vi "cube vision timed.vi"() -> ()   [LabVIEW 2017]
uses:
  <vilib>/vision/NI_Vision_Development_Module.lvlib
panel:
  out "trim image":u32=1
  out "fps":dbl=40.0
  out "total time":u32=25
  out "to 3D array":u32=6
  out "calc angle":u32
  out "threshhold":u32
  out "isolate green":u32=18
  out "to RGB array":u32=1
  out "angle":dbl=-14.305551846621954
  out "Color":T1(plugin-control)
  out "Binary Image":T1(plugin-control)
  in  "Sat Range":cluster{u8, u8}(slide)={255, 160} scale=0.0..255.0
  in  "Hue Range":cluster{u8, u8}(slide)={87, 19} scale=0.0..255.0
  in  "File Path":path=path "F:/power cube pics/5.bmp"
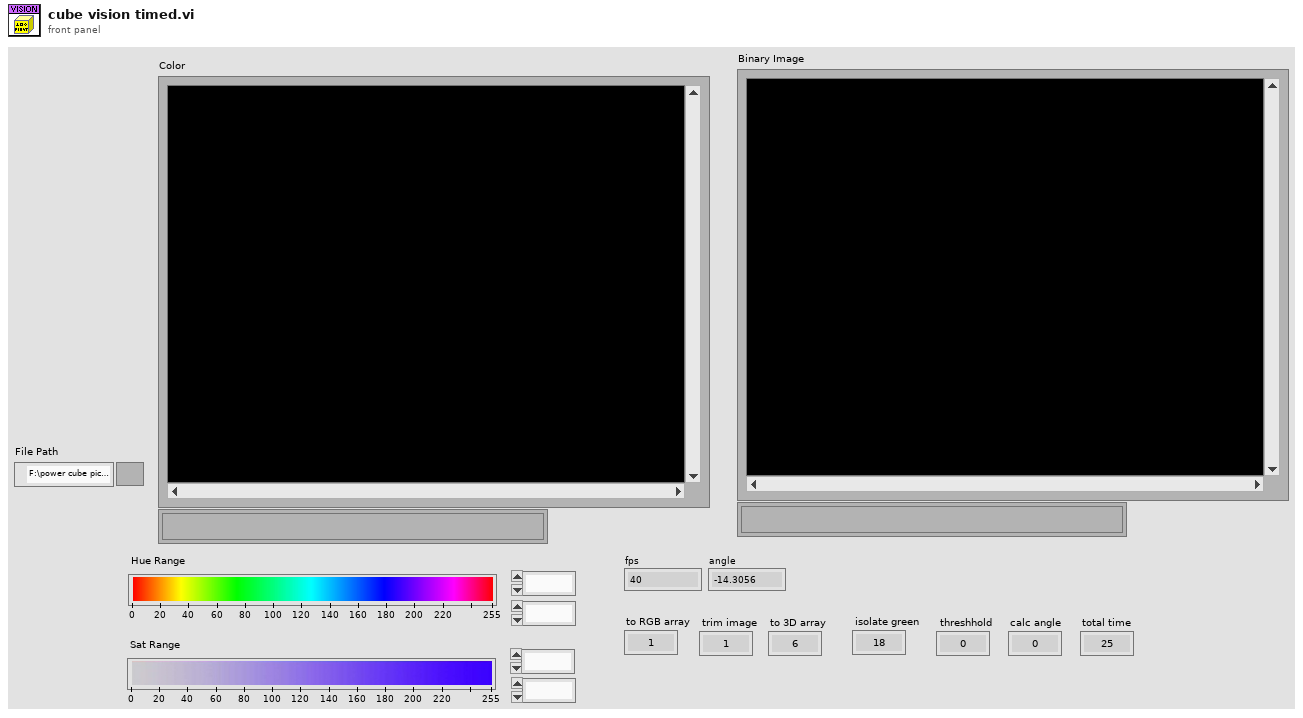
[diagram p1: front panel]
types:
  T1 = typedef "IMAQ Image.ctl" = refnum<image>
  T2 = typedef "Image Type" = u32
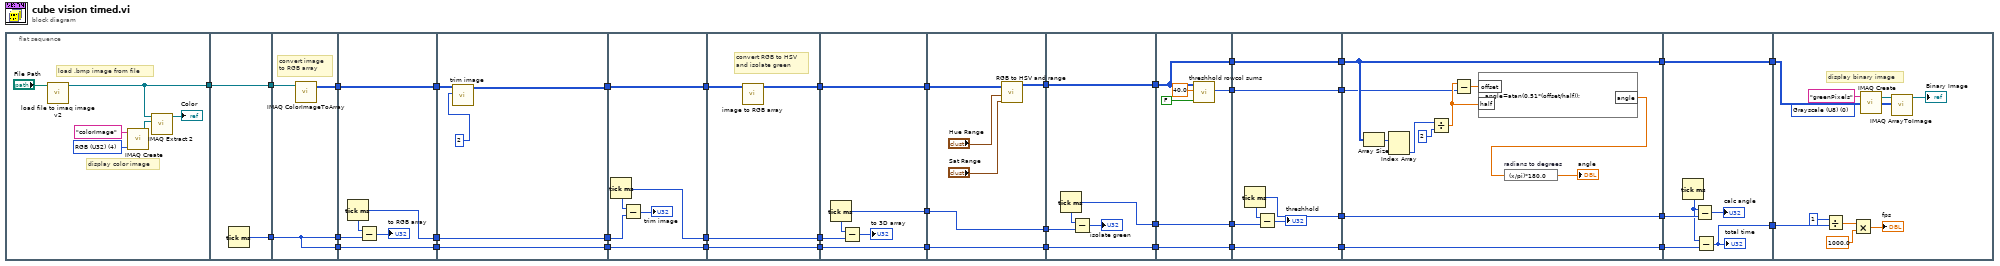
[diagram p0: block diagram]
diagram:
  n1 = flat-sequence {
    tunnel: [w42] -> w40
    tunnel: w40 -> [w48]
    tunnel: [w48] -> w39
    tunnel: [w47] -> w29
    tunnel: w39 -> [w51]
    tunnel: [w50] -> w38
    tunnel: [w49] -> w30
    tunnel: w29 -> [w49]
    tunnel: [w49] -> w18
    tunnel: w38 -> [w56]
    tunnel: [w56] -> w9
    tunnel: w30 -> [w55]
    tunnel: [w53] -> w8
    tunnel: w18 -> [w52]
    tunnel: [w52] -> w7
    tunnel: w9 -> [w59]
    tunnel: [w57] -> w6
    tunnel: w8 -> [w61]
    tunnel: [w61] -> w4
    tunnel: w7 -> [w60]
    tunnel: [w60] -> w2
    tunnel: w6 -> [w66]
    tunnel: [w66] -> w5
    tunnel: w4 -> [w63]
    tunnel: [w62] -> w3
    tunnel: w2 -> [w65]
    tunnel: [w65] -> w1
    tunnel: w5 -> [w70]
    tunnel: [w69] -> w22
    tunnel: w3 -> [w68]
    tunnel: [w68] -> w21
    tunnel: w1 -> [w67]
    tunnel: [w67] -> w17
    tunnel: [w75] -> w23
    tunnel: w22 -> [w75]
    tunnel: w21 -> [w73]
    tunnel: [w72] -> w19
    tunnel: w17 -> [w71]
    tunnel: [w71] -> w16
    tunnel: [w79] -> w24
    tunnel: w23 -> [w78]
    tunnel: [w77] -> w20
    tunnel: w19 -> [w77]
    tunnel: w16 -> [w76]
    tunnel: [w76] -> w15
    tunnel: w24 -> [w86]
    tunnel: [w86] -> w37
    tunnel: [w84] -> w27
    tunnel: w20 -> [w83]
    tunnel: w15 -> [w82]
    tunnel: [w82] -> w14
    tunnel: w37 -> [w92]
    tunnel: [w92] -> w36
    tunnel: [w89] -> w34
    tunnel: [w88] -> w28
    tunnel: w27 -> [w88]
    tunnel: w14 -> [w87]
    tunnel: [w87] -> w13
    tunnel: w36 -> [w98]
    tunnel: [w98] -> w35
    tunnel: w34 -> [w97]
    tunnel: [w97] -> w33
    tunnel: w28 -> [w95]
    tunnel: [w94] -> w26
    tunnel: w13 -> [w93]
    tunnel: [w93] -> w12
    tunnel: w35 -> [w109]
    tunnel: w33 -> [w104]
    tunnel: [w109] -> w32
    tunnel: w26 -> [w100]
    tunnel: [w100] -> w25
    tunnel: w12 -> [w99]
    tunnel: [w99] -> w11
    tunnel: w32 -> [w115]
    tunnel: [w115] -> w31
    tunnel: w25 -> [w113]
    tunnel: w11 -> [w111]
    tunnel: [w110] -> w10
    tunnel: w31 -> [w121]
    tunnel: w10 -> [w120]
    frame #0 {
      w44 = T2 4 items=["Grayscale (U8)", "Grayscale (I16)", "Grayscale (SGL)", "Complex (CSG)", "RGB (U32)", "HSL (U32)", "RGB (U64)", "Grayscale (U16)"] ("Image Type")
      # "display color image"
      # "load .bmp image from file"
      n2 = call "load file to imaq image v2.vi"("path to BMP file"="File Path") -> ("Image"=w42:T1)  [unwired: 9 in, 1 out]
      n3 = call "IMAQ Create"("Image Name"="colorImage", "Image Type"=w44) -> ("New Image"=w46:T1)  [unwired: 3 in, 1 out]
      n4 = call "IMAQ Extract 2"("Image Dst"=w46, "Image Src"=w42) -> ("Image Dst Out"=→"Color":T1)  [unwired: 8 in, 1 out]
    }
    frame #1 {
      n5 = Tick Count (ms)() -> (millisecond timer value=w47:u32)
    }
    frame #2 {
      # "convert image\nto RGB array"
      n6 = call "IMAQ ColorImageToArray"("Image"=w51) -> ("Image Pixels (U32)"=w50:u32[][])  [unwired: 3 in, 2 out]
    }
    frame #3 {
      n7 = Tick Count (ms)() -> (millisecond timer value=w53:u32)
      n8 = Subtract(x=w53, y=w55) -> (x-y=→"to RGB array":u32)
    }
    frame #4 {
      n9 = call "trim image.vi"("scale"=2, "Image Pixels (U32)"=w59) -> ("Trimmed Image Pixels (U32)"=w57:u32[][])  [unwired: 9 in]
    }
    frame #5 {
      n10 = Tick Count (ms)() -> (millisecond timer value=w62:u32)
      n11 = Subtract(x=w62, y=w63) -> (x-y=→"trim image":u32)
    }
    frame #6 {
      # "convert RGB to HSV\nand isolate green"
      n12 = call "image to RGB array.vi"("Image Pixels (U32)"=w70) -> ("Image Pixels (U8)"=w69:u8[][][])  [unwired: 10 in]
    }
    frame #7 {
      n13 = Tick Count (ms)() -> (millisecond timer value=w72:u32)
      n14 = Subtract(x=w72, y=w73) -> (x-y=→"to 3D array":u32)
    }
    frame #8 {
      n15 = call "RGB to HSV and range.vi"("Image Pixels (RGB)"=w78, "Hue Range"="Hue Range", "Sat Range"="Sat Range") -> ("Threshholded Pixels"=w79:u8[][])  [unwired: 7 in]
    }
    frame #9 {
      n16 = Tick Count (ms)() -> (millisecond timer value=w84:u32)
      n17 = Subtract(x=w84, y=w83) -> (x-y=→"isolate green":u32)
    }
    frame #10 {
      n18 = call "threshhold rowcol sums.vi"("Row(T)/Col(F)"=FALSE, "Threshold"=40.0, "Pixels"=w92) -> ("middle row/col"=w89:i32)  [unwired: 6 in, 2 out]
    }
    frame #11 {
      n19 = Tick Count (ms)() -> (millisecond timer value=w94:u32)
      n20 = Subtract(x=w94, y=w95) -> (x-y=→"threshhold":u32)
    }
    frame #12 {
      n21 = Array Size(array=w109) -> (size(s)=w105:i32[])
      n22 = Index Array(array=w105) -> (element #2=w106:i32)  [unwired: 2 in, 1 out]
      n23 = Divide(x=w106, y=2) -> (x/y=w108:dbl)
      n24 = Subtract(x=w108, y=w104) -> (x-y=w107:dbl)
      n25 = formula code="angle=atan(0.51*(offset/half));"("offset"=w107, "half"=w108) -> ("angle"=w101:dbl)
      n26 = expression code="(x/pi)*180.0" "radians to degrees"(w101) -> (→"angle":dbl)
    }
    frame #13 {
      n27 = Tick Count (ms)() -> (millisecond timer value=w112:u32)
      n28 = Subtract(x=w112, y=w113) -> (x-y=→"calc angle":u32)
      n29 = Subtract(x=w112, y=w111) -> (x-y=w110:u32)
      "total time" <- w110
    }
    frame #14 {
      (unwired) T2 0 items=["Grayscale (U8)", "Grayscale (I16)", "Grayscale (SGL)", "Complex (CSG)", "RGB (U32)", "HSL (U32)", "RGB (U64)", "Grayscale (U16)"] ("Image Type")
      # "display binary image"
      n30 = Divide(x=u32 1, y=w120) -> (x/y=w118:dbl)
      n31 = Multiply(x=w118, y=1000.0) -> (x*y=→"fps":dbl)
      n32 = call "IMAQ Create"("Image Name"="greenPixels") -> ("New Image"=w123:T1)  [unwired: 4 in, 1 out]
      n33 = call "IMAQ ArrayToImage"("Image Pixels (U8)"=w121, "Image"=w123) -> ("Image Out"=→"Binary Image":T1)  [unwired: 8 in, 1 out]
    }
  }
